vi "String Pot 2016.vi"(7 "Array in":refnum<k24>[](array[refnum]), 8 "error in (no error)":errorcluster, 9 "Descriptions":string[](array[string]), 10 "String Pot \nSlope":dbl=1.7339999675750732 format="%.2f", 11 "Sensor Cluster":T1) -> (0 "error out":errorcluster, 2 "Sensor Cluster 2":T1, 3 "Distance (in)":dbl format="%.2f", 5 "Array out":refnum<k24>[](array[refnum]))   [LabVIEW 2016]
uses:
  Waterloo DAQ/controls/MCC DAQ Readings.ctl
  C:/Program Files (x86)/National Instruments/LabVIEW 2016/vi.lib/ULx/ULx_LV.dll
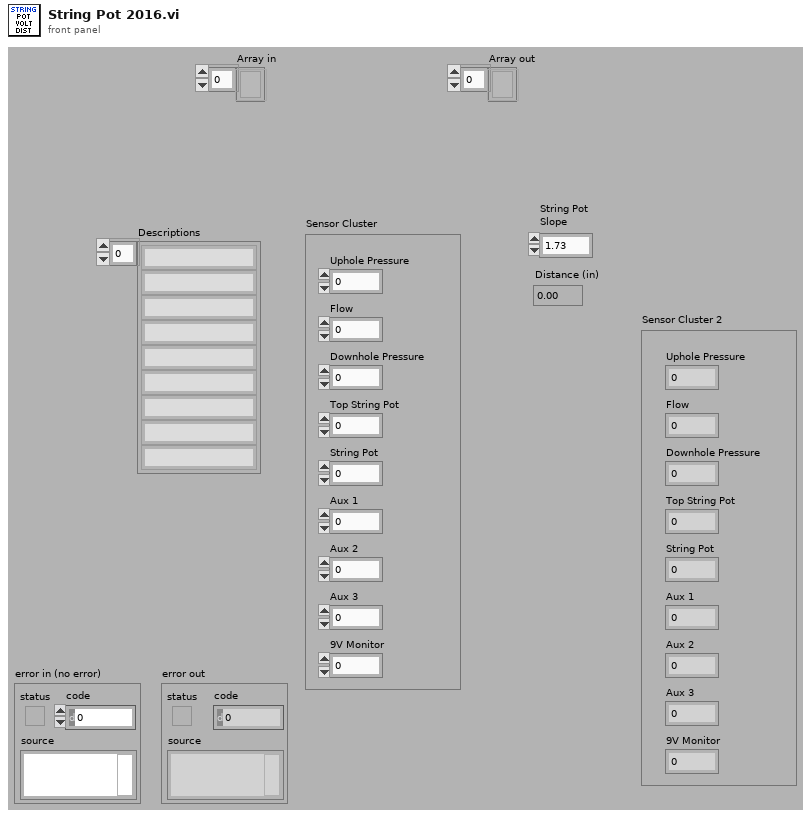
[diagram p1: front panel]
types:
  T1 = typedef "MCC DAQ Readings.ctl" = cluster{"Uphole Pressure":dbl, "Flow":dbl, "Downhole Pressure":dbl, "Top String Pot":dbl, "String Pot":dbl, "Aux 1":dbl, "Aux 2":dbl, "Aux 3":dbl, "9V Monitor":dbl}
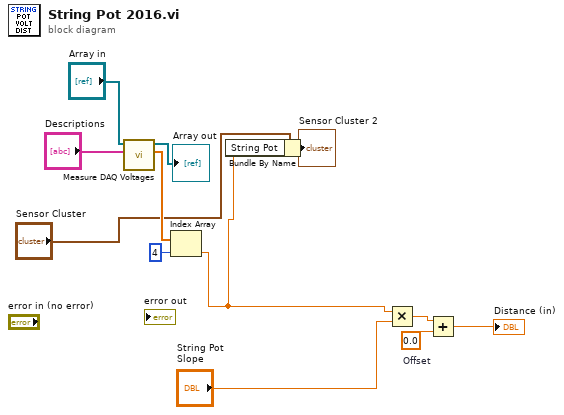
[diagram p0: block diagram]
diagram:
  w11 = 0.0  # Offset
  n1 = call "Measure DAQ Voltages.vi"("Descriptions"="Descriptions", "Array in"="Array in") -> ("Raw Voltages"=w4:dbl[], "Array out"=→"Array out":refnum<k24>[])  [unwired: 7 in, 1 out]
  n2 = Index Array(array=w4, index=4) -> (element=w2:dbl)
  n3 = Bundle By Name(cluster="Sensor Cluster", "String Pot"=w2) -> (→"Sensor Cluster 2":T1)
  n4 = Multiply(x=w2, y="String Pot \nSlope") -> (x*y=w12:dbl)
  n5 = Add(x=w12, y=w11) -> (x+y=→"Distance (in)":dbl)
